vi "Create data.vi"(8 "error in (no error)":errorcluster, 11 "Example Class A in":refnum<class "ExampleClassA.lvclass">) -> (0 "error out":errorcluster, 2 "Graph":dbl[](graph), 3 "Example Class A out":refnum<class "ExampleClassA.lvclass">)   [LabVIEW 2012, in "ExampleClassA.lvclass"]
doc: "Creates noisy sinus data."
uses:
  ExampleClassA.lvclass
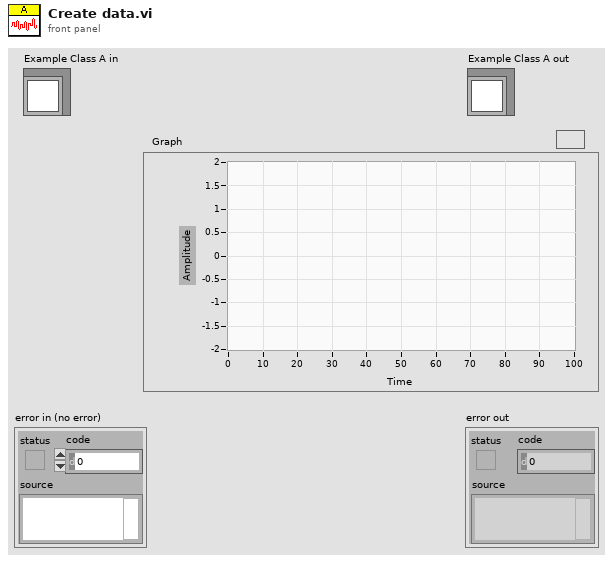
[diagram p1: front panel]
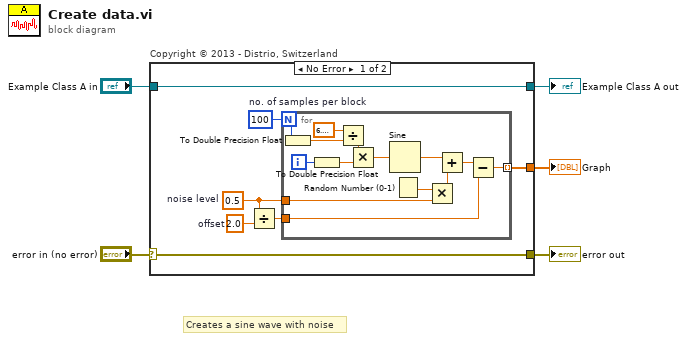
[diagram p0: block diagram]
diagram:
  # "Creates a sine wave with noise"
  n1 = case "Copyright © 2013 - Distrio, Switzerland" shown="No Error" "error in (no error)" {
    selector: "error in (no error)" -> [w6 w28]
    tunnel: [w6 w28] -> w4
    tunnel: [w12 w27] -> w2
    tunnel: "Example Class A in" -> [w12 w27]
    tunnel: [w7 _] -> w1
    frame No Error {
      w10 = 2.0  # offset
      w8 = 0.5  # noise level
      w11 = 100  # no. of samples per block
      n2 = Divide(x=w8, y=w10) -> (x/y=w9:dbl)
      n3 = for {
        N: w11 -> [w25]
        tunnel: [w13] -> w7 mode=indexing
        tunnel: w9 -> [w16]
        tunnel: w8 -> [w15]
        i -> [w23]
        n4 = To Double Precision Float(number=w25) -> (double precision float=w22:dbl)
        n5 = To Double Precision Float(number=w23) -> (double precision float=w21:dbl)
        n6 = Divide(x=6.283185307179586, y=w22) -> (x/y=w24:dbl)
        n7 = Multiply(x=w24, y=w21) -> (x*y=w20:dbl)
        n8 = Sine(x=w20) -> (sin(x)=w17:dbl)
        n9 = Random Number (0-1)() -> (number: 0 to 1=w19:dbl)
        n10 = Multiply(x=w19, y=w15) -> (x*y=w18:dbl)
        n11 = Add(x=w17, y=w18) -> (x+y=w14:dbl)
        n12 = Subtract(x=w14, y=w16) -> (x-y=w13:dbl)
      }
    }
    frame Error {
    }
  }
  "error out" <- w4
  "Example Class A out" <- w2
  "Graph" <- w1
